vi "net_var_loop.vi"(8 "error in":errorcluster) -> (0 "error out":errorcluster)   [LabVIEW 2010]
uses:
  <vilib>/Platform/TimedLoop/XDataNode/XDataNode.xnode
  <vilib>/Platform/TimedLoop/XDataNode/timing_clust.ctl
  <vilib>/Platform/TimedLoop/XDataNode/nitl_modes.ctl
  <vilib>/Platform/TimedLoop/XDataNode/wakeup.ctl
  initialization/micron_globals.vi
  <vilib>/Analysis/baseanly.llb/A x Vector.vi
  <vilib>/Platform/TimedLoop/XDataNode/XDNodeRunTimeDep.lvlib
  <vilib>/Analysis/NI_AALBase.lvlib
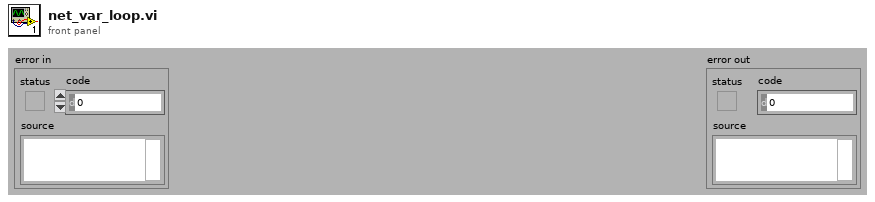
[diagram p1: front panel]
types:
  T1 = typedef "XDNodeRunTimeDep.lvlib/timing_clust.ctl" = cluster{"Expected End [f-1]":u64, "Actual End [f-1]":u64, "Finished Late? [f-1]":bool, "Expected End [i-1]":u64, "Actual End [i-1]":u64, "Finished Late? [i-1]":bool, "Expected Start [i]":u64, "Actual Start [i]":u64, "Expected Start [f]":u64, "Actual Start [f]":u64, "Source Name":string, "Structure Name":string, "Period":i64, "Deadline":i64, "Offset":i64, "Start":i64, "Priority":i32, "Timeout":i32, "Mode":T2, "Wakeup Reason":T3, "Error":errorcluster, "Source Type":string, "Secondary Source Type":string, "Global End Time":u64, "Global Start Time":u64, "Frame Duration":u64, "Iteration Duration":u64, "Assigned CPU":i32, "I/O Scan Engine Mode":u32}
  T2 = typedef "XDNodeRunTimeDep.lvlib/nitl_modes.ctl" = enum32{"No Change", "Process missed periods, maintain original phase", "Discard missed periods, maintain original phase", "Process missed periods, ignore original phase", "Discard missed periods, ignore original phase"}
  T3 = typedef "XDNodeRunTimeDep.lvlib/wakeup.ctl" = enum32{"Normal", "Aborted", "Asynchronous wakeup", "Timing source error", "Timed loop error", "Timeout"}
  T4 = typedef "NI_Matrix.lvlib/RealMatrix.ctl" = dbl[][]
  T5 = typedef "Micron params.ctl" = cluster{"Stimulus":T6, "Goal Filter A":T8, "Mode controls":T9, "Manipulator type":enum16{"Current piezo", "Voltage piezo"}, "Manipulator calibration":T10, "Network":T12, "Goal Filter B":T8, "Cancellation":T13, "Transition time":sgl, "Estimation and Feedforward":cluster{"Use Raw Data (ignore Kalman Filter)":bool, "Turn Kalman Filter Off":bool, "Use IMC (if off, PID is used)":bool, "KP":sgl, "KI":sgl, "KD":sgl, "Feedforward Control":bool, "Velocity Gain":dbl[], "KF input delay":i32}}
  T6 = typedef "stimulus.ctl" = cluster{"Type":enum16{"Off", "Step", "Sine", "Triangle", "Arbitrary"}, "Delay":i32, "Amplitude":sgl[], "Injection point":T7, "Closed loop":bool, "Offset":sgl[], "Tip -> world":bool}
  T7 = typedef "injection_point.ctl" = enum16{"Total pose", "V limiter", "Goal ", "Inverse kin", "Controller", "Output", "DAC"}
  T8 = typedef "goal_filter_parms.ctl" = cluster{"Lower Fc":sgl, "Lower Q":sgl, "Scale factor":sgl, "Upper Fc":sgl, "Upper Q":sgl, "Manip zeroing":sgl, "Speedup max":sgl, "Speedup thresh":sgl, "Speedup nonlin":sgl, "V limit":sgl, "V limit range":sgl}
  T9 = typedef "mode_conrols.ctl" = cluster{"Hold":bool, "Cancellation":bool, "Goal filter":bool, "Trigger":bool}
  T10 = typedef "manipulator_cal.ctl" = cluster{"Tip offset":sgl[], "Tip light calibration":T11, "Axial filter":cluster{"filter structure":enum32{"IIR 2nd Order", "IIR 4th Order"}, "Reverse Coefficients":dbl[], "Forward Coefficients":dbl[]}, "Lateral filter":cluster{"filter structure":enum32{"IIR 2nd Order", "IIR 4th Order"}, "Reverse Coefficients":dbl[], "Forward Coefficients":dbl[]}, "Handle light calibration":T11, "RCM offset":sgl[], "Base pivots":sgl[][], "Output pivots":sgl[][], "Length center":sgl}
  T11 = typedef "probe_calibration.ctl" = sgl[][]
  T12 = typedef "network_params.ctl" = cluster{"Remote Host":string, "Send Status":bool, "Send Port":u16, "Recv Commands":bool, "Recv Port":u16}
  T13 = typedef "im_control_params.ctl" = cluster{"Bandwidth":sgl, "Delay":i32, "Stack travel":sgl, "Saturation pos":sgl, "Slew Limit":sgl, "Turnoff zeroing":sgl, "Bypass":bool}
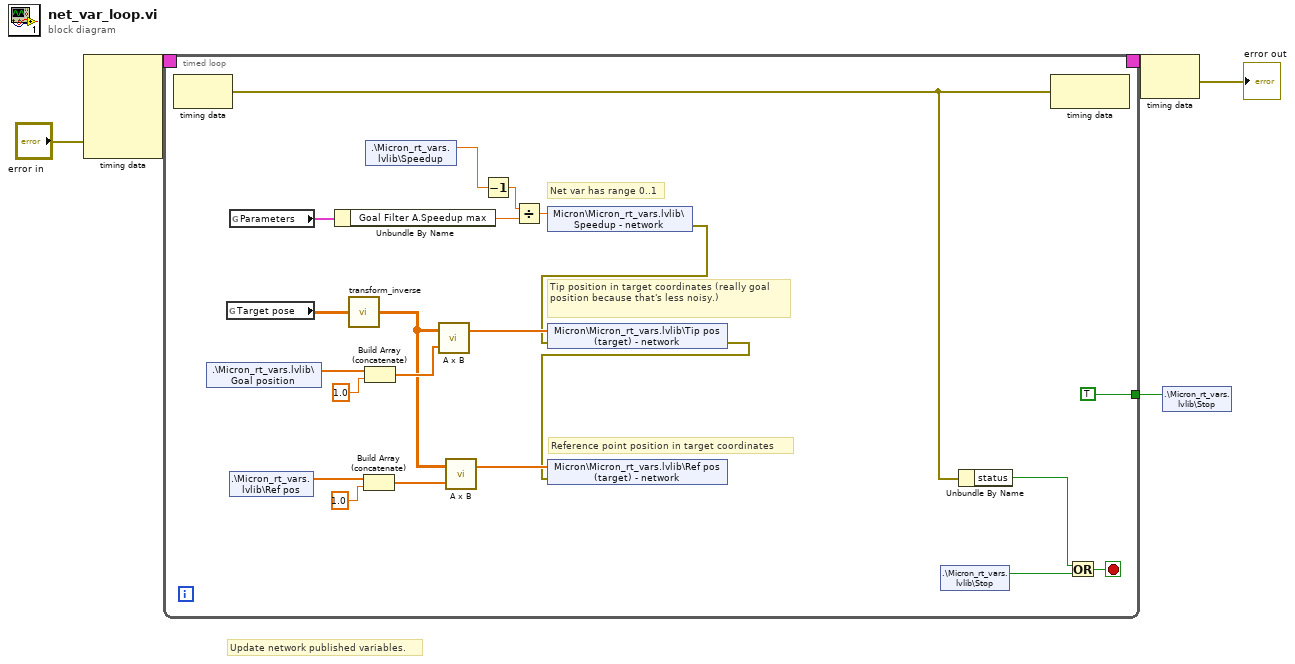
[diagram p0: block diagram]
diagram:
  # "Update network published variables."
  n1 = node-c288("error in") -> (w5:T1)  [unwired: 4 out]
  n2 = timed-loop {
    timing: w5 -> [_]
    timing-out: [_] -> w4
    tunnel: [TRUE ("stop - RT")] -> w1
    stop <- w10 stop-if-true
    # "Reference point position in target coordinates"
    # "Tip position in target coordinates (really goal position because that's less noisy.)"
    # "Net var has range 0..1"
    n3 = node-c288() -> (w6:errorcluster)  [unwired: 1 out]
    n4 = shared-variable ".\\Micron_rt_vars.lvlib\\Goal position"() -> (w22:sgl[])  [unwired: 2 out]
    n5 = global read "micron_globals.vi" "Target pose"() -> (w19:T4)
    n6 = global read "micron_globals.vi" "Parameters"() -> (w27:T5)
    n7 = shared-variable ".\\Micron_rt_vars.lvlib\\Ref pos"() -> (w14:sgl[])  [unwired: 2 out]
    n8 = Unbundle By Name(w27) -> ("Goal Filter A.Speedup max"=w25:sgl)
    n9 = call "transform_inverse.vi"("Transform"=w19) -> ("Inverse transform"=w16:T4)
    n10 = Build Array (concatenate)(w14, sgl 1.0) -> (w13:sgl[])
    n11 = Build Array (concatenate)(w22, sgl 1.0) -> (w20:sgl[])
    n12 = shared-variable ".\\Micron_rt_vars.lvlib\\Speedup"() -> (w24:sgl)  [unwired: 2 out]
    n13 = call-poly <vilib>:"A x B.vi"("Vector"=w20, "A"=w16) -> ("A x Vector"=w18:dbl[])  [unwired: 1 out]
    n14 = call-poly <vilib>:"A x B.vi"("Vector"=w13, "A"=w16) -> ("A x Vector"=w17:dbl[])  [unwired: 1 out]
    n15 = Decrement(x=w24) -> (x-1=w23:sgl)
    n16 = Divide(x=w23, y=w25) -> (x/y=w26:sgl)
    n17 = shared-variable "Micron\\Micron_rt_vars.lvlib\\Speedup - network"(w26) -> (error out=w12:errorcluster)  [unwired: 1 out]
    n18 = shared-variable "Micron\\Micron_rt_vars.lvlib\\Tip pos (target) - network"(w18, error in=w12) -> (error out=w11:errorcluster)
    n19 = shared-variable "Micron\\Micron_rt_vars.lvlib\\Ref pos (target) - network"(w17, error in=w11) -> ()  [unwired: 1 out]
    n20 = shared-variable ".\\Micron_rt_vars.lvlib\\Stop"() -> (w9:bool)  [unwired: 2 out]
    n21 = Unbundle By Name(w6) -> ("status"=w8:bool)
    n22 = node-c288(w6) -> ()  [unwired: 1 out]
    n23 = Or(x=w8, y=w9) -> (x .or. y?=w10:bool)
  }
  n24 = node-c288(w4) -> (→"error out":errorcluster)
  n25 = shared-variable ".\\Micron_rt_vars.lvlib\\Stop"(w1) -> ()  [unwired: 2 out]
